vi "Active.vi"(8 "error in (no error)":errorcluster, 10 "Message In":refnum<class "Message.lvclass">, 11 "System Actor in":refnum<class "System Actor.lvclass">) -> (0 "error out":errorcluster, 3 "System Actor out":refnum<class "System Actor.lvclass">)   [LabVIEW 2024, in "System Actor.lvclass"]
uses:
  System Actor.lvclass
  System Actor.lvclass/System Actor.ctl
  Message/Message.lvclass
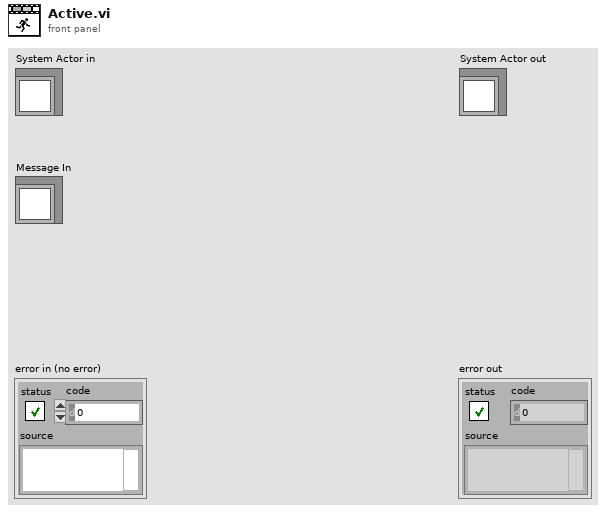
[diagram p1: front panel]
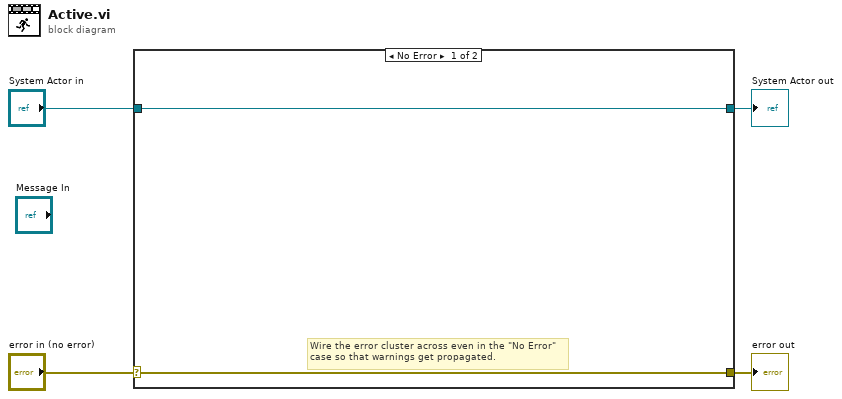
[diagram p0: block diagram]
diagram:
  n1 = case shown="No Error" "error in (no error)" {
    selector: "error in (no error)" -> [w5 w8]
    tunnel: [w5 w8] -> w3
    tunnel: [w6 w7] -> w1
    tunnel: "System Actor in" -> [w6 w7]
    frame No Error {
      # "Wire the error cluster across even in the \"No Error\"\ncase so that warnings get propagated."
    }
    frame Error {
    }
  }
  "error out" <- w3
  "System Actor out" <- w1
